vi "EAGLE GUI V4.vi"() -> ()   [LabVIEW 2015]
panel:
  in  "Save Button 2":bool
  in  "Save Button":bool
  out "Table Control":string[][](table)
  out "Iris Found Status":bool
  out "Image":T1(plugin-control)
  in  "Previous":bool
  in  "Tab":enum32{"Page 1", "Page 2", "Page 3", "Page 4"}(tab)
  in  "EditRoute":bool
  in  "Next":bool
  # "Immediate Actions"
  # "Patient Info"
  # "Using the Joystick: Aim the pupil to the center of the Cross,\nMerage the two Focus Beams, \nClick next when ready to start a new procedure."
  # "Instructions"
  # "Instructions"
  # "IRIS FOUND!\nIn order to Edit the Iris Border click EDIT.\nClick Next when ready"
  # "Instructions"
  # "READY FOR CLINICAL ACTIONS\nClick next to start the procedure"
  # "Instructions"
  # "CLINICAL ACTIONS ARE TAKING PLACE\nWait for finish"
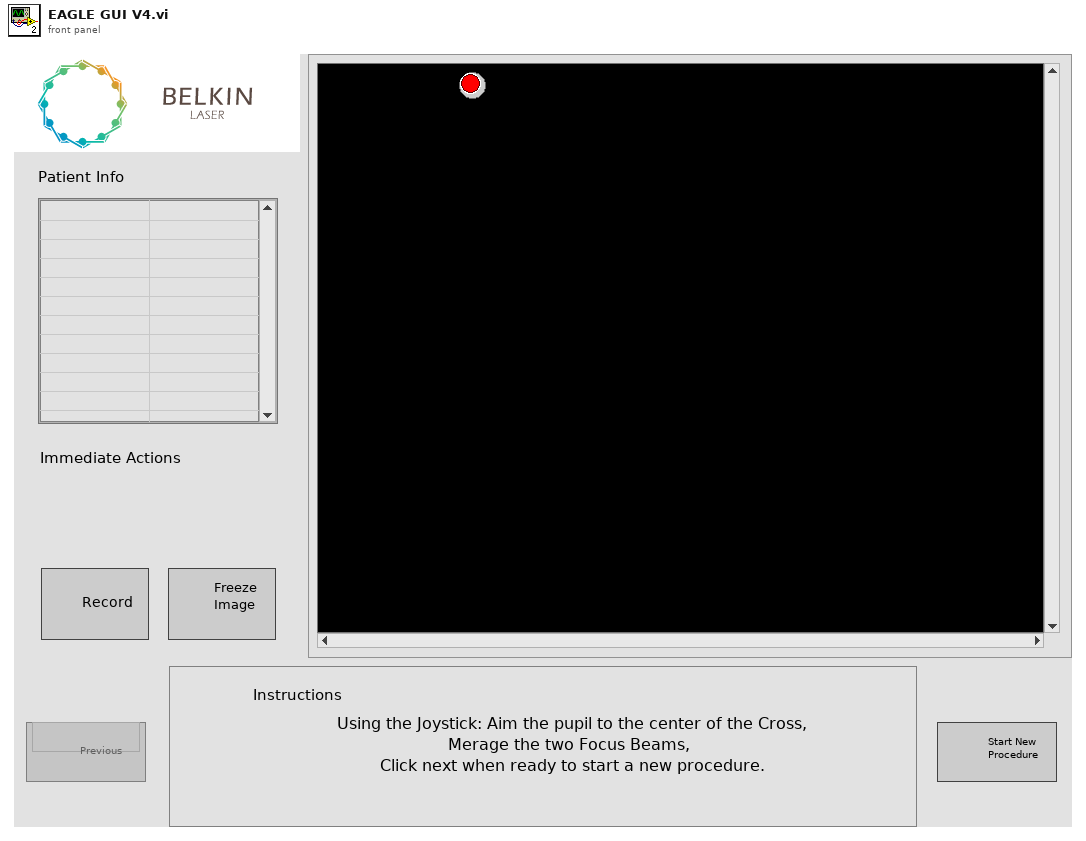
[diagram p1: front panel]
types:
  T1 = typedef "IMAQ Image.ctl" = refnum<image>
  T2 = enum8{"Enabled", "Disabled", "Disabled and Grayed Out"}
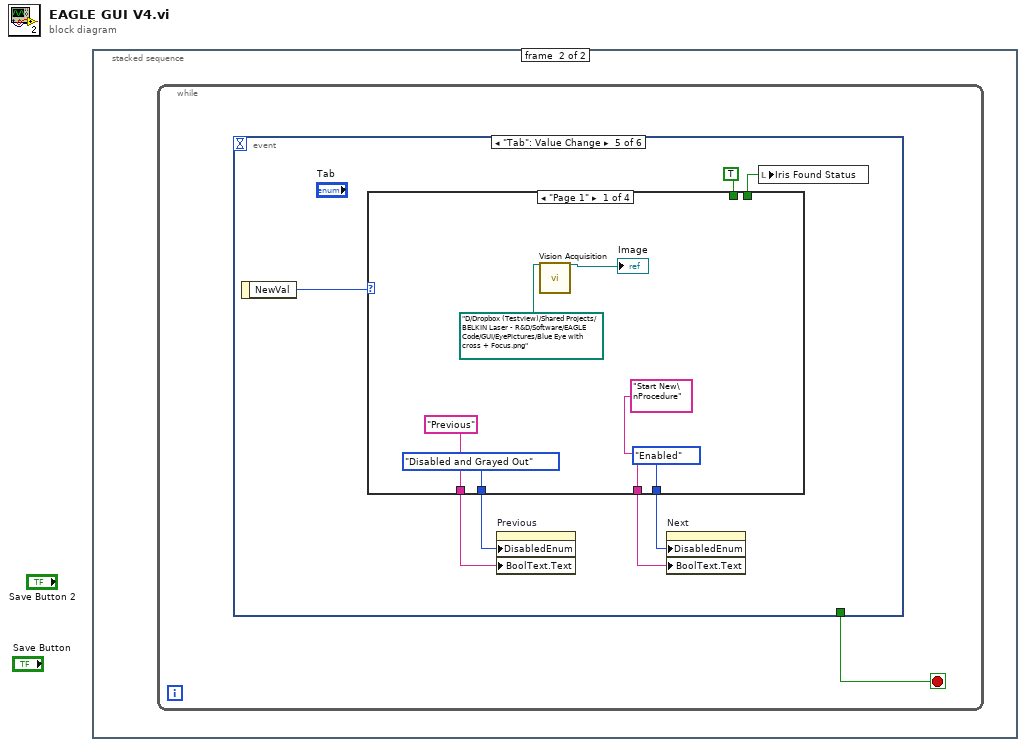
[diagram p0: block diagram]
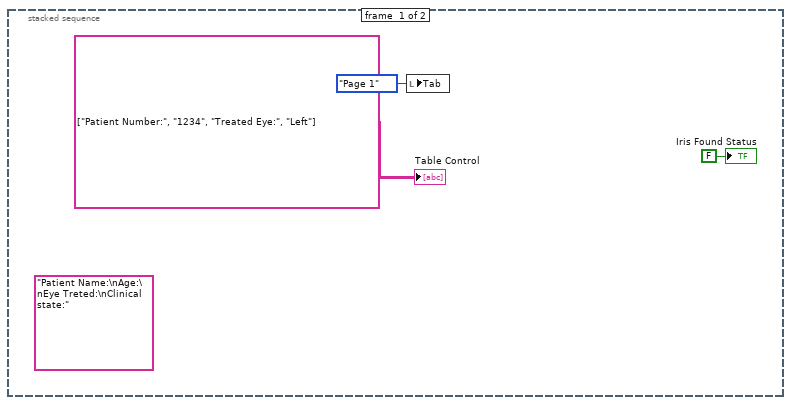
[diagram p2: hidden frame]
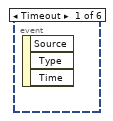
[diagram p3: hidden frame]
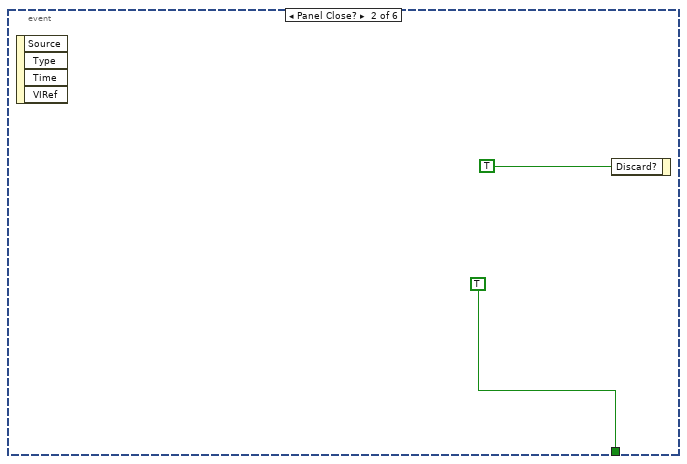
[diagram p4: hidden frame]
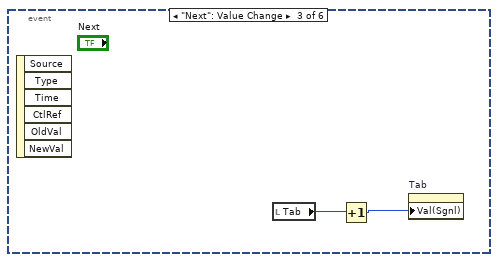
[diagram p5: hidden frame]
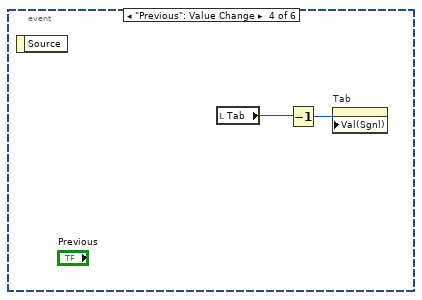
[diagram p6: hidden frame]
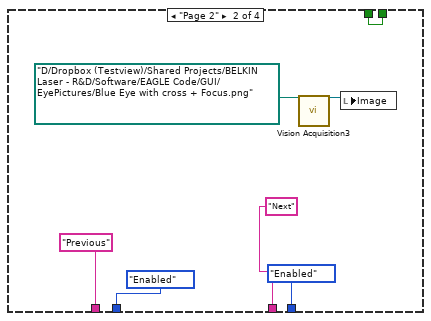
[diagram p7: hidden frame]
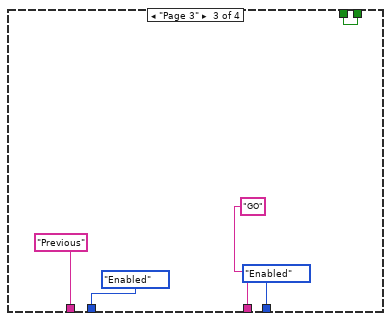
[diagram p8: hidden frame]
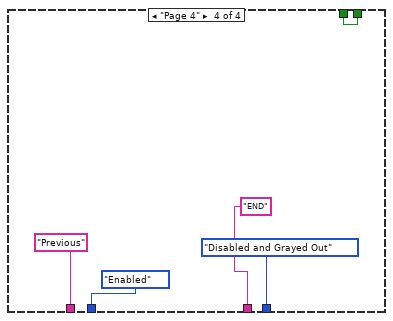
[diagram p9: hidden frame]
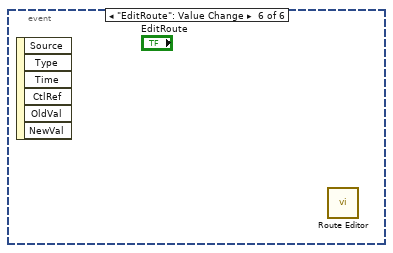
[diagram p10: hidden frame]
diagram:
  n1 = stacked-sequence {
    frame #0 {
      (unwired) "Patient Name:\nAge:\nEye Treted:\nClinical state:" ("patient Info")
      n2 = local write "Tab"(enum32{"Page 1", "Page 2"}."Page 1" ("Tab")) -> ()
      "Table Control" <- string[][] [["Patient Number:", "1234"], ["Treated Eye:", "Left"]] ("Table Control")
      "Iris Found Status" <- FALSE ("Iris Found Status")
    }
    frame #1 {
      n3 = while {
        stop <- w4 stop-if-true
        n4 = event shown="[4] \"Tab\": Value Change" {
          selector: _ -> [_ _ _ _ _ _]
          dyn-events: _ -> [_ _ _ _ _ _]
          timeout: _ -> [_ _ _ _ _ _]
          tunnel: [_ TRUE _ _ _ _] -> w4
          event Timeout {
            n5 = event-data() -> ()  [unwired: 1 in, 3 out]
          }
          event Panel Close? {
            n6 = event-data() -> ()  [unwired: 1 in, 4 out]
            n7 = event-data("Discard?"=TRUE) -> ()  [unwired: 1 in, 1 out]
          }
          event "Next": Value Change {
            n8 = event-data() -> ()  [unwired: 1 in, 6 out]
            n9 = local read "Tab"() -> (w7:enum32{"Page 1", "Page 2", "Page 3", "Page 4"})
            n10 = Increment(x=w7) -> (x+1=w8:enum32{"Page 1", "Page 2", "Page 3", "Page 4"})
            n11 = property on="Tab" class="TabCtl (strict)"("Val(Sgnl)"=w8) -> ()  [unwired: 2 in, 2 out]
          }
          event "Previous": Value Change {
            n12 = event-data() -> ()  [unwired: 1 in, 1 out]
            n13 = local read "Tab"() -> (w10:enum32{"Page 1", "Page 2", "Page 3", "Page 4"})
            n14 = Decrement(x=w10) -> (x-1=w9:enum32{"Page 1", "Page 2", "Page 3", "Page 4"})
            n15 = property on="Tab" class="TabCtl (strict)"("Val(Sgnl)"=w9) -> ()  [unwired: 2 in, 2 out]
          }
          event "Tab": Value Change {
            n16 = event-data() -> ("NewVal"=w17:enum32{"Page 1", "Page 2", "Page 3", "Page 4"})  [unwired: 1 in]
            n17 = case shown="\"Page 1\"" w17 {
              tunnel: [T2."Disabled and Grayed Out" ("Disabled") T2."Enabled" ("Disabled") T2."Enabled" ("Disabled") T2."Enabled" ("Disabled")] -> w16
              tunnel: [T2."Enabled" ("Disabled") T2."Enabled" ("Disabled") T2."Enabled" ("Disabled") T2."Disabled and Grayed Out" ("Disabled")] -> w15
              tunnel: ["Start New\nProcedure" "Next" "GO" "END"] -> w14
              tunnel: ["Previous" "Previous" "Previous" "Previous"] -> w13
              tunnel: [_ w24 w31 w36] -> w12
              tunnel: TRUE -> [_ w24 w31 w36]
              frame "Page 1" {
                n18 = call "Vision Acquisition"("Image Path"=path "D:/Dropbox (Testview)/Shared Projects/BELKIN Laser - R&D/Software/EAGLE Code/GUI/EyePictures/Blue Eye with cross + Focus.png") -> ("Image Out"=→"Image":T1)  [unwired: 25 in, 1 out]
              }
              frame "Page 2" {
                n19 = call "Vision Acquisition3"("Image Path"=path "D:/Dropbox (Testview)/Shared Projects/BELKIN Laser - R&D/Software/EAGLE Code/GUI/EyePictures/Blue Eye with cross + Focus.png") -> ("Image Out"=w26:T1)  [unwired: 25 in, 1 out]
                n20 = local write "Image"(w26) -> ()
              }
              frame "Page 3" {
              }
              frame "Page 4" {
              }
            }
            n21 = property on="Previous" class="Bool"("DisabledEnum"=w16, "BoolText.Text"=w13) -> ()  [unwired: 2 in, 2 out]
            n22 = property on="Next" class="Bool"("DisabledEnum"=w15, "BoolText.Text"=w14) -> ()  [unwired: 2 in, 2 out]
            n23 = local write "Iris Found Status"(w12) -> ()
          }
          event "EditRoute": Value Change {
            n24 = event-data() -> ()  [unwired: 1 in, 6 out]
            n25 = call "Route Editor.vi"() -> ()  [unwired: 11 in, 1 out]
          }
        }
      }
    }
  }
